vi "Render Partial.vi"(6 "Loader":refnum<class "Loader.lvclass">, 8 "Error In":errorcluster, 10 "Partial":refnum<class "Partial.lvclass">, 11 "Context In":refnum<class "Context.lvclass">) -> (0 "Error Out":errorcluster, 2 "Output":string, 3 "Context Out":refnum<class "Context.lvclass">)   [LabVIEW 2018, in "Toolkit.lvlib"]
uses:
  Toolkit.lvlib
  Nodes/Partial/Partial.lvclass
  Context/Context.lvclass
  Loaders/Loader/Loader.lvclass
  Nodes/Partial/Partial.lvclass/Partial.ctl
  Lex String.vi
  Nodes/Root/Root.lvclass
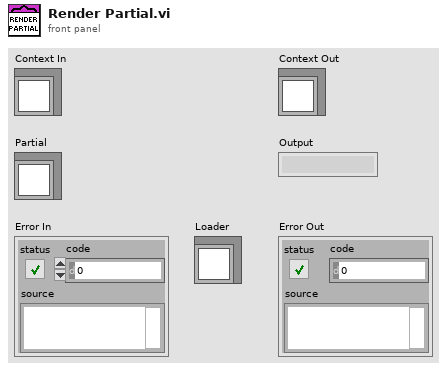
[diagram p1: front panel]
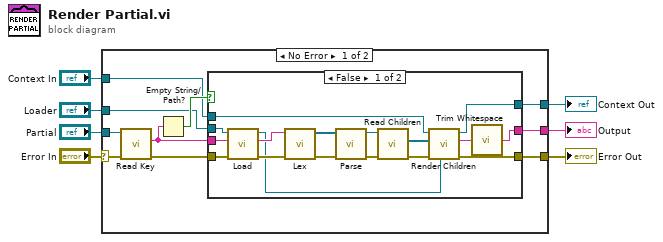
[diagram p0: block diagram]
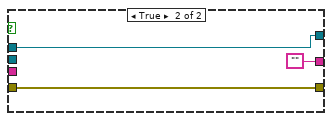
[diagram p2: hidden frame]
diagram:
  n1 = case shown="No Error" "Error In" {
    selector: "Error In" -> [w16 w38]
    tunnel: "Partial" -> [w17 _]
    tunnel: [w10 w38] -> w6
    tunnel: [w12 w39] -> w5
    tunnel: "Context In" -> [w13 w39]
    tunnel: [w14 _] -> w2
    tunnel: "Loader" -> [w9 _]
    frame No Error {
      n2 = call "Read Key.vi"("Error In"=w16, "Partial In"=w17) -> ("Error Out"=w11:errorcluster, "Key"=w8:string)  [unwired: 7 in, 1 out]
      n3 = Empty String/Path?(string/path=w8) -> (empty?=w15:bool)
      n4 = case shown="False" w15 {
        tunnel: [w18 ""] -> w14
        tunnel: w13 -> [w24 w36]
        tunnel: [w23 w36] -> w12
        tunnel: w11 -> [w32 w35]
        tunnel: [w22 w35] -> w10
        tunnel: w9 -> [w34 _]
        tunnel: w8 -> [w33 _]
        frame False {
          n5 = call-dynamic "Load.vi"("Error In"=w32, "Key"=w33, "Loader In"=w34) -> ("Error Out"=w30:errorcluster, "Template"=w31:string, "Loader Out"=w21:refnum<class "Loader.lvclass">)  [unwired: 6 in]
          n6 = call-poly "Lex.vi"("Error In"=w30, "Input"=w31) -> ("Error Out"=w28:errorcluster, "Tokens"=w29:refnum<class "Token.lvclass">[])  [unwired: 8 in]
          n7 = call "Parse.vi"("Error In"=w28, "Tokens"=w29) -> ("Error Out"=w26:errorcluster, "Abstract Syntax Tree"=w27:refnum<class "Root.lvclass">)  [unwired: 8 in]
          n8 = call-dynamic "Read Children.vi"("Error In"=w26, "Non-Terminal In"=w27) -> ("Error Out"=w20:errorcluster, "Children"=w25:refnum<class "Node.lvclass">[])  [unwired: 7 in, 1 out]
          n9 = call "Render Children.vi"("Loader"=w21, "Error In"=w20, "Children"=w25, "Context In"=w24) -> ("Error Out"=w22:errorcluster, "Output"=w19:string, "Context Out"=w23:refnum<class "Context.lvclass">)  [unwired: 5 in]
          n10 = call <vilib>:"Trim Whitespace.vi"("string"=w19) -> ("trimmed string"=w18:string)  [unwired: 1 in]
        }
        frame True {
        }
      }
    }
    frame Error {
    }
  }
  "Error Out" <- w6
  "Output" <- w2
  "Context Out" <- w5
